vi "FilterOthersExceptFile.vi"(11 "Array in":T1[](array[typedef])) -> (3 "Array out":T1[](array[typedef]))   [LabVIEW 2014]
uses:
  FTP Toolkit/FTP Class/controls/Dir-File Info.ctl
  FTP Toolkit/FTP Class/controls/Dir-File Type.ctl
  FTP Toolkit/FTP Class/FTP.lvclass
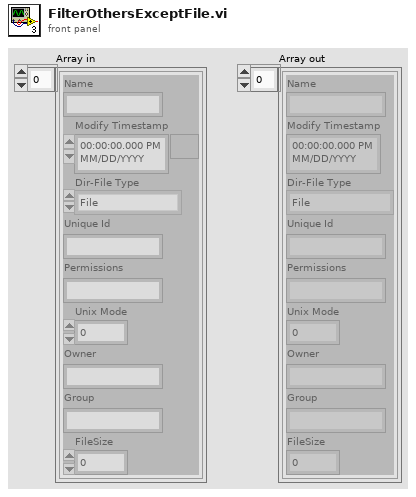
[diagram p1: front panel]
types:
  T1 = typedef "FTP.lvlib/FTP.lvclass/Dir-File Info.ctl" = cluster{"Name":string, "Modify Timestamp":timestamp, "Dir-File Type":T2, "Unique Id":string, "Permissions":string, "Unix Mode":u16, "Owner":string, "Group":string, "FileSize":i64}
  T2 = typedef "FTP.lvlib/FTP.lvclass/Dir-File Type.ctl" = enum16{"File", "Listed Directory", "Parent Directory", "Directory", "Unknown"}
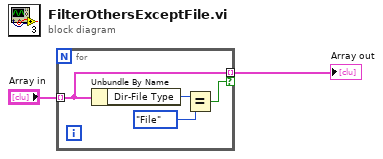
[diagram p0: block diagram]
diagram:
  n1 = for {
    tunnel: "Array in" -> [w3] mode=indexing
    tunnel: [w3] -> w2 mode=indexing if=w4
    n2 = Unbundle By Name(w3) -> ("Dir-File Type"=w6:T2)
    n3 = Equal?(x=w6, y=Dir-File_Type."File") -> (x = y?=w4:bool)
  }
  "Array out" <- w2
